vi "set_file_name_base.vi"(8 "error in (no error)":errorcluster, 10 "file name base":string, 11 "GenericComponent in":refnum<class "GenericComponent.lvclass">) -> (0 "error out":errorcluster, 3 "GenericComponent out":refnum<class "GenericComponent.lvclass">)   [LabVIEW 2010, in "GenericComponent.lvclass"]
uses:
  GenericComponent.lvclass
  class_data.vi
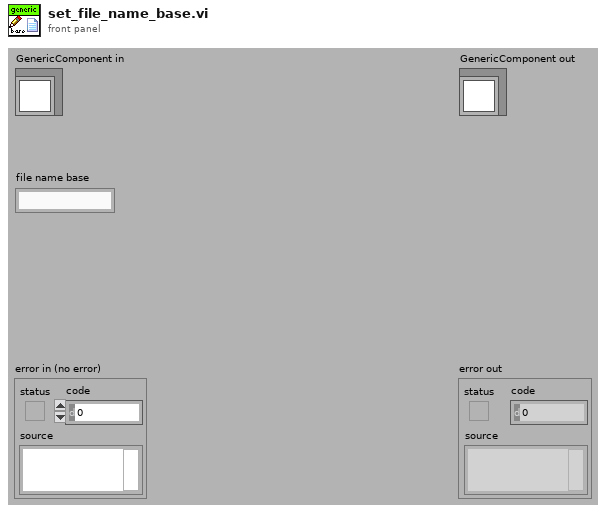
[diagram p1: front panel]
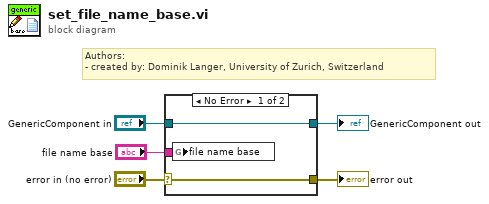
[diagram p0: block diagram]
diagram:
  # "Authors: \n- created by: Dominik Langer, University of Zurich, Switzerland"
  n1 = case shown="No Error" "error in (no error)" {
    selector: "error in (no error)" -> [w7 w10]
    tunnel: [w7 w10] -> w4
    tunnel: [w8 w9] -> w2
    tunnel: "GenericComponent in" -> [w8 w9]
    tunnel: "file name base" -> [w6 _]
    frame No Error {
      n2 = global write "class_data.vi" "file name base"(w6) -> ()
    }
    frame Error {
    }
  }
  "error out" <- w4
  "GenericComponent out" <- w2
